vi "readU64FIFO.vi"(8 "error in (no error)":errorcluster, 9 "Timeout":i32, 10 "NumberOfElements":u32, 11 "IReadU64FIFO in":refnum<class "IReadU64FIFO.lvclass">) -> (0 "error out":errorcluster, 1 "ElementsRemaining":u32, 2 "Data":u64[](array[numeric]), 3 "IReadU64FIFO out":refnum<class "IReadU64FIFO.lvclass">)   [LabVIEW 2016, in "RTFPGA.lvlib" / "IReadU64FIFO.lvclass"]
uses:
  IReadU64FIFO.lvclass
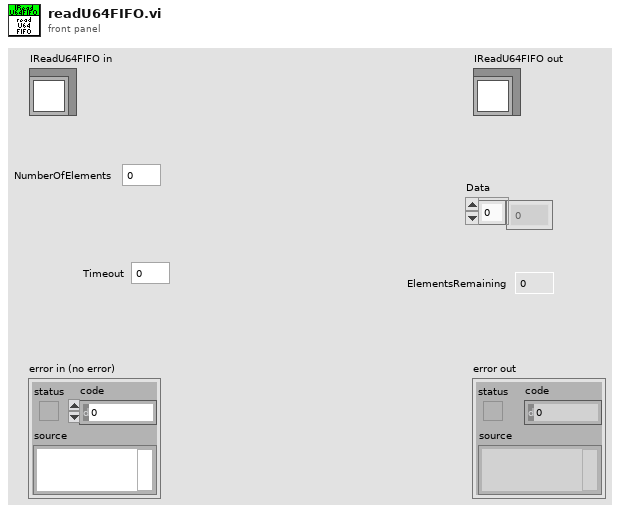
[diagram p1: front panel]
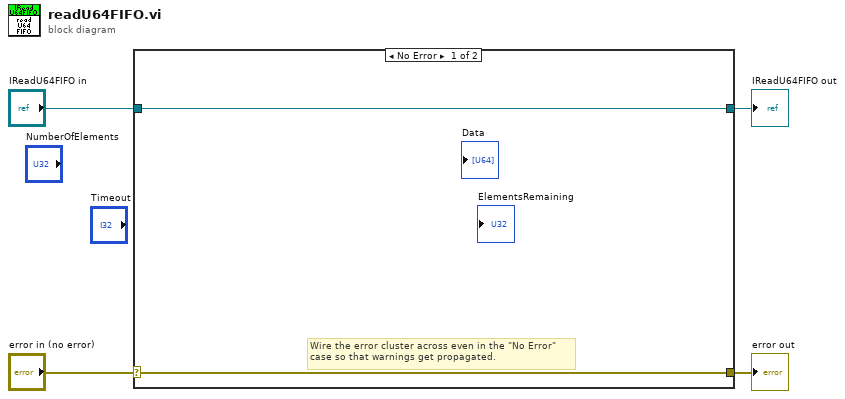
[diagram p0: block diagram]
diagram:
  n1 = case shown="No Error" "error in (no error)" {
    selector: "error in (no error)" -> [w5 w8]
    tunnel: [w5 w8] -> w3
    tunnel: [w6 w7] -> w1
    tunnel: "IReadU64FIFO in" -> [w6 w7]
    frame No Error {
      # "Wire the error cluster across even in the \"No Error\"\ncase so that warnings get propagated."
    }
    frame Error {
    }
  }
  "error out" <- w3
  "IReadU64FIFO out" <- w1
